vi "Subvi AO.vi"(8 "AO in":u16, 9 "Nmax":u32, 10 "Memory label":refnum<k21>="AO1 buffer", 11 "AO channel":refnum<k21>="Connector1/AO0") -> (0 "AO out":u16)   [LabVIEW 2017]
uses:
  <vilib>/rvi/Emulation/niFpgaGetClockAttributes.vi
  <vilib>/rvi/Emulation/niFpgaSctlEmulationGetInTimedLoop.vi
  <vilib>/rvi/Emulation/niFpgaEmulationReportErrorSimple.vi
  <vilib>/rvi/eio/common/nirviEmuTemplateMethod_errors.vi
  <vilib>/rvi/DataTransferAndStorage/Container/Common/niFpgaContainerExecOnDevCompGetState.vi
  <vilib>/rvi/Emulation/niFpgaEmulationIsFPGAContextNoSignature.vi
  <vilib>/rvi/DataTransferAndStorage/Container/Common/niFpgaContainerGetUniqueNameForEmu.vi
  <vilib>/rvi/Emulation/niFpgaProcessEmulError.vi
  <vilib>/rvi/errors/nirviReportUnexpectedCaseInternalError (U32).vi
  <vilib>/rvi/Memory/Memory_Emulation/niFpgaMemoryEmulationCacheClearOnFirstRun.vi
  <vilib>/rvi/Memory/Memory_Emulation/nirvimemoryEmulationManagerCache_MakeExclusive.vi
  <vilib>/rvi/Memory/Memory_Emulation/niFpgaMemoryEmulationValidateCache.vi
  <vilib>/rvi/Memory/Memory_Emulation/nirvimemoryEmulationManagerCache_InsertValue.vi
  <vilib>/Utility/error.llb/Clear Errors.vi
  <vilib>/rvi/Memory/Memory_Emulation/nirvimemoryEmulationManagerCache_ReleaseExclusive.vi
  <vilib>/rvi/Memory/Memory_Emulation/nirvimemoryEmulationManagerCache_GetValue.vi
  <vilib>/rvi/Memory/Memory_Emulation/nirvimemoryEmulationManagerCache_SetValue.vi
  <vilib>/rvi/Emulation/niFpgaSctlEmulationResourceMgr.vi
  <vilib>/rvi/Emulation/niFpgaCriticalErrorInLSC.vi
  GV trigger.vi
  <vilib>/eio/EIONode/EIONode.xnode
  <vilib>/rvi/DataTransferAndStorage/Container/XNode/niFpgaContainer.xnode
  <vilib>/rvi/Memory/Memory_Emulation/niFpgaMemoryEmulationRefIn.vi
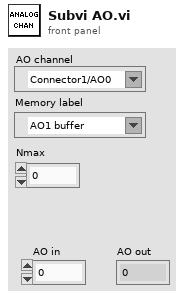
[diagram p1: front panel]
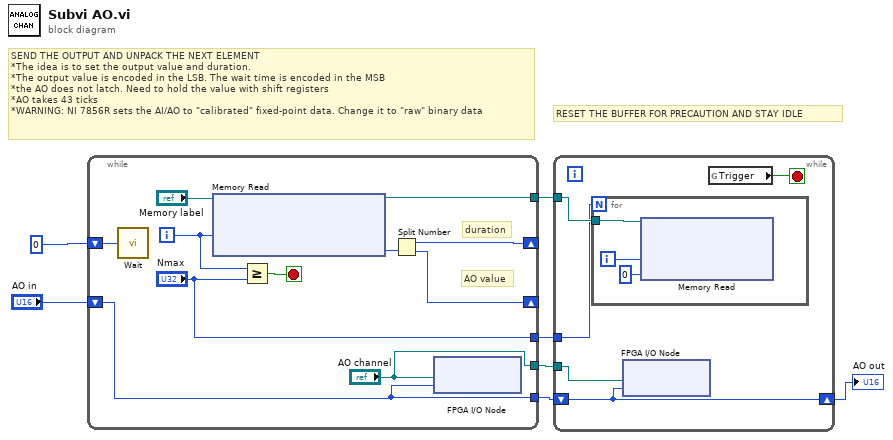
[diagram p0: block diagram]
diagram:
  # "RESET THE BUFFER FOR PRECAUTION AND STAY IDLE"
  # "SEND THE OUTPUT AND UNPACK THE NEXT ELEMENT\n*The idea is to set the output value and duration.\n*The output value is encoded in the LSB. The wait time is encoded in the MSB\n*the AO does not latch. Need to hold the value with shift registers\n*AO takes 43 ticks\n*WARNING: NI 7856R sets the AI/AO to \"calibrated\" fixed-point data. Change it to \"raw\" binary data"
  n1 = while {
    shift-right: [w17] -> _
    shift-left: u16 0 -> [w18]
    shift-right: [w15] -> _
    shift-left: "AO in" -> [w13]
    tunnel: [w13] -> w5
    tunnel: ["AO channel"] -> w3
    tunnel: [w11] -> w2
    tunnel: ["Nmax"] -> w1
    i -> [w12]
    stop <- w14 stop-if-true
    # "duration"
    # "AO value"
    n2 = call "Wait"("Count(Ticks)"=w18) -> ()  [unwired: 1 out]
    n3 = xnode ("Memory Read")("Memory In"="Memory label", "Address"=w12) -> ("Memory Out"=w11:refnum<k21>, "Data"=w16:u32)
    n4 = Greater Or Equal?(x=w12, y="Nmax") -> (x >= y?=w14:bool)
    n5 = Split Number(x=w16) -> (hi(x)=w17:u16, lo(x)=w15:u16)
    n6 = xnode "FPGA I/O Node"("I/O Item"=w13, "FPGA I/O In"="AO channel") -> ()  [unwired: 1 out]
  }
  n7 = while {
    shift-right: [w21] -> w4
    shift-left: w5 -> [w21]
    tunnel: w3 -> [w22]
    tunnel: w2 -> [w20]
    tunnel: w1 -> [w19]
    stop <- w23 stop-if-true
    n8 = for {
      N: w19 -> [_]
      tunnel: w20 -> [w26]
      i -> [w24]
      n9 = xnode ("Memory Read")("Address"=w24, "Data"=u32 0, "Memory In"=w26) -> ()  [unwired: 1 out]
    }
    n10 = xnode "FPGA I/O Node"("I/O Item"=w21, "FPGA I/O In"=w22) -> ()  [unwired: 1 out]
    n11 = global read "GV trigger.vi" "Trigger"() -> (w23:bool)
  }
  "AO out" <- w4
